vi "AssetMgrCreateDeviceFromHardwareResponse_Create.vi"(7 "Header":T16, 8 "error in (no error)":errorcluster, 9 "ResponseError":errorcluster, 10 "AssetMgrCreateDeviceFromHardwareResponse":T1, 11 "IRoutingSource":T15) -> (0 "error out":errorcluster, 3 "Message":T17)   [LabVIEW 2017]
uses:
  <vilib>/addons/InsightCM/MessageBus/Base/controls/Message.ctl
  <vilib>/addons/InsightCM/MessageBus/Base/controls/MessageHeader.ctl
  <vilib>/addons/InsightCM/MessageBus/Base/controls/KeyValuePair.ctl
  <vilib>/addons/InsightCM/MessageBus/Base/controls/IRoutingSource.ctl
  <vilib>/addons/InsightCM/MessageBus/MessageLibrary/AssetManager/controls/AssetMgrCreateDeviceFromHardwareResponseBody.ctl
  <vilib>/addons/InsightCM/MessageBus/Base/controls/DeviceModel.ctl
  <vilib>/addons/InsightCM/MessageBus/Base/controls/Device.ctl
  <vilib>/addons/InsightCM/MessageBus/Base/controls/DeviceState.ctl
  <vilib>/addons/InsightCM/MessageBus/Base/controls/DataGroup.ctl
  <vilib>/addons/InsightCM/MessageBus/Base/controls/BurstModeTrigger.ctl
  <vilib>/addons/InsightCM/MessageBus/Base/controls/Trigger.ctl
  <vilib>/addons/InsightCM/MessageBus/Base/controls/Condition.ctl
  <vilib>/addons/InsightCM/MessageBus/Base/controls/DeviceSensorGroup.ctl
  <vilib>/addons/InsightCM/MessageBus/Base/controls/WirelessEndpoint.ctl
  <vilib>/addons/InsightCM/MessageBus/Base/controls/WirelessChannel.ctl
  <vilib>/addons/InsightCM/MessageBus/Base/controls/Channel.ctl
  <vilib>/addons/InsightCM/MessageBus/Base/controls/Tag.ctl
  <vilib>/addons/InsightCM/MessageBus/Base/controls/MessageClassType.ctl
  <vilib>/addons/InsightCM/Utilities/PropertyHelpers/PropertyHelpers.lvlib
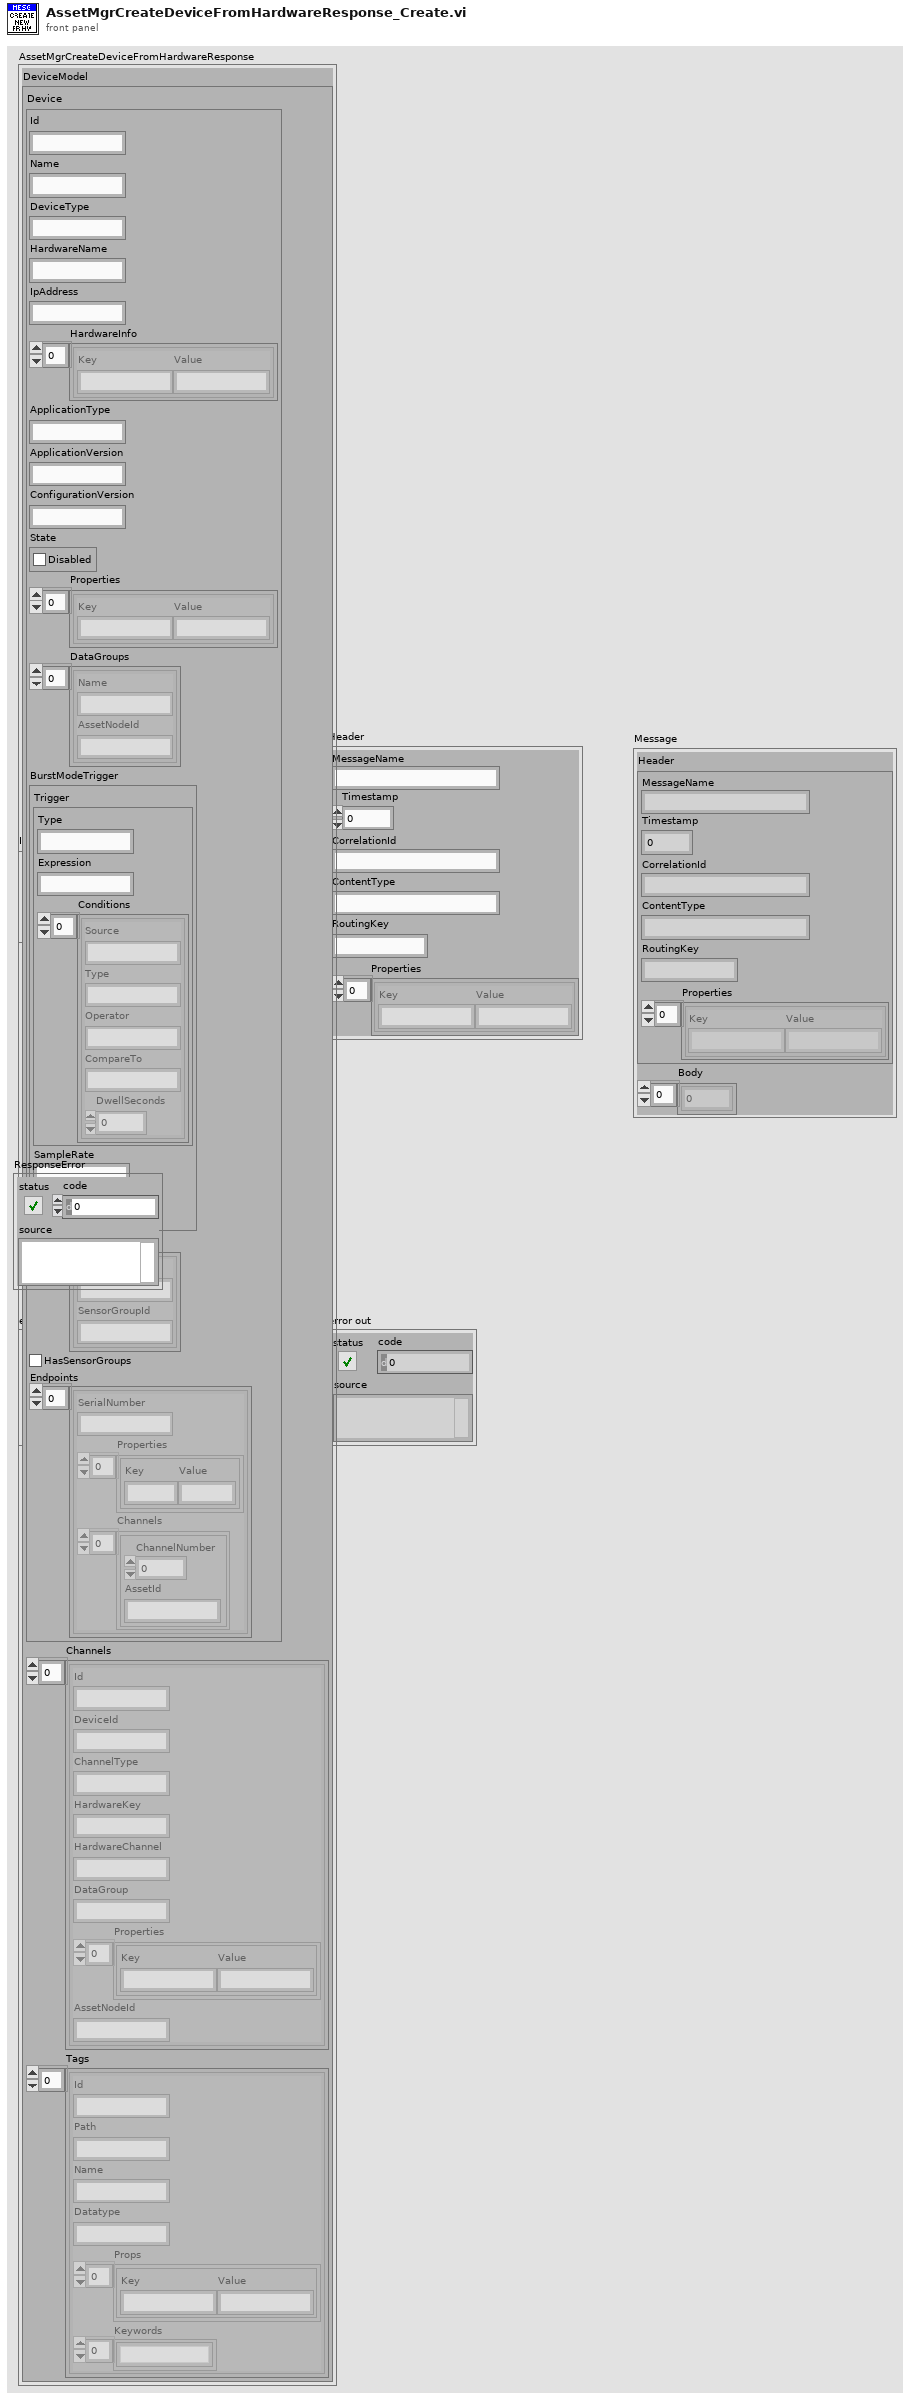
[diagram p1: front panel]
types:
  T1 = typedef "AssetMgrCreateDeviceFromHardwareResponseBody.ctl" = cluster{"DeviceModel":T2}
  T2 = typedef "DeviceModel.ctl" = cluster{"Device":T3, "Channels":T13[], "Tags":T14[]}
  T3 = typedef "Device.ctl" = cluster{"Id":string, "Name":string, "DeviceType":string, "HardwareName":string, "IpAddress":string, "HardwareInfo":T4[], "ApplicationType":string, "ApplicationVersion":string, "ConfigurationVersion":string, "State":T5, "Properties":T4[], "DataGroups":T6[], "BurstModeTrigger":T7, "SensorGroups":T10[], "HasSensorGroups":bool, "Endpoints":T11[]}
  T4 = typedef "KeyValuePair.ctl" = cluster{"Key":string, "Value":string}
  T5 = typedef "DeviceState.ctl" = cluster{"Disabled":bool}
  T6 = typedef "DataGroup.ctl" = cluster{"Name":string, "AssetNodeId":string}
  T7 = typedef "BurstModeTrigger.ctl" = cluster{"Trigger":T8, "SampleRate":string, "AcquisitionLength":string}
  T8 = typedef "Trigger.ctl" = cluster{"Type":string, "Expression":string, "Conditions":T9[]}
  T9 = typedef "Condition.ctl" = cluster{"Source":string, "Type":string, "Operator":string, "CompareTo":string, "DwellSeconds":dbl}
  T10 = typedef "DeviceSensorGroup.ctl" = cluster{"EquipId":string, "SensorGroupId":string}
  T11 = typedef "WirelessEndpoint.ctl" = cluster{"SerialNumber":string, "Properties":T4[], "Channels":T12[]}
  T12 = typedef "WirelessChannel.ctl" = cluster{"ChannelNumber":i32, "AssetId":string}
  T13 = typedef "Channel.ctl" = cluster{"Id":string, "DeviceId":string, "ChannelType":string, "HardwareKey":string, "HardwareChannel":string, "DataGroup":string, "Properties":T4[], "AssetNodeId":string}
  T14 = typedef "Tag.ctl" = cluster{"Id":string, "Path":string, "Name":string, "Datatype":string, "Props":T4[], "Keywords":string[]}
  T15 = typedef "IRoutingSource.ctl" = cluster{"CorrelationId":string, "ReplyTo":string}
  T16 = typedef "MessageHeader.ctl" = cluster{"MessageName":string, "Timestamp":i64, "CorrelationId":string, "ContentType":string, "RoutingKey":string, "Properties":T4[]}
  T17 = typedef "Message.ctl" = cluster{"Header":T16, "Body":u8[]}
  T18 = typedef "MessageClassType.ctl" = enum16{"Request", "Response", "Broadcast", "RoutedMessage"}
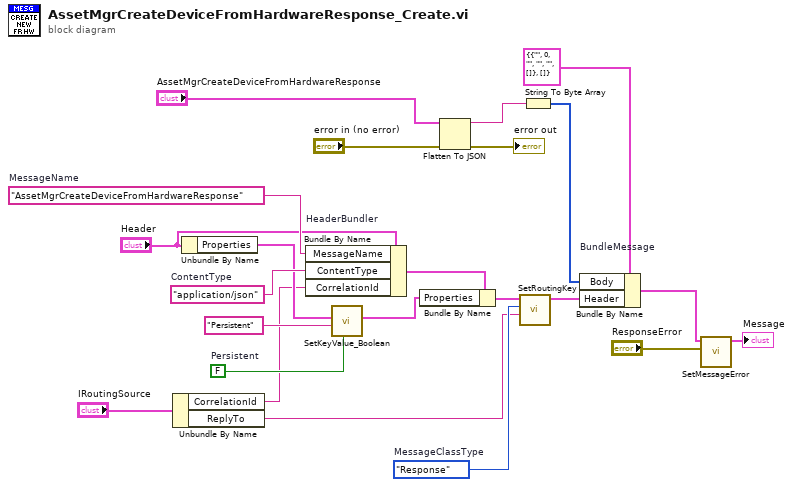
[diagram p0: block diagram]
diagram:
  w19 = MessageClassType."Response"  # MessageClassType
  w14 = FALSE  # Persistent
  w20 = "AssetMgrCreateDeviceFromHardwareResponse"  # MessageName
  w17 = "application/json"  # ContentType
  n1 = Unbundle By Name("IRoutingSource") -> ("CorrelationId"=w4:string, "ReplyTo"=w3:string)
  n2 = Unbundle By Name("Header") -> ("Properties"=w16:T4[])
  n3 = Bundle By Name "HeaderBundler"(cluster="Header", "MessageName"=w20, "ContentType"=w17, "CorrelationId"=w4) -> (w11:T16)
  n4 = call <vilib>:"SetKeyValue_Boolean.vi"("value"=w14, "key"="Persistent" ("Key"), "key value pairs"=w16) -> ("key value pairs out"=w10:T4[])  [unwired: 8 in]
  n5 = Bundle By Name(cluster=w11, "Properties"=w10) -> (w12:T16)
  n6 = Flatten To JSON(anything="AssetMgrCreateDeviceFromHardwareResponse", error in (no error)="error in (no error)") -> (JSON string=w2:string, 11:→"error out":errorcluster)  [unwired: 1 in]
  n7 = call <vilib>:"SetRoutingKey.vi"("SendTo"=w3, "MessageClassType"=w19, "Message Header in"=w12) -> ("Message Header out"=w13:T16)  [unwired: 8 in]
  n8 = String To Byte Array(string=w2) -> (unsigned byte array=w22:u8[])
  n9 = Bundle By Name "BundleMessage"(cluster=T17 {"Header"={"MessageName"="", "Timestamp"=0, "CorrelationId"="", "ContentType"="", "RoutingKey"="", "Properties"=[]}, "Body"=[]} ("Message"), "Body"=w22, "Header"=w13) -> (w8:T17)
  n10 = call <vilib>:"SetMessageError.vi"("error"="ResponseError", "message in"=w8) -> ("message out"=→"Message":T17)  [unwired: 9 in]
